vi "Choo Choo Test Bench.vi"() -> ()   [LabVIEW 2013]
doc: "This VI imlements the framework and scheduler for your robotics program. It should not be necessary to modify the framework. You are expected to add your code to the VIs called from Robot Main, the ones located in the Team Code within the project."
uses:
  <vilib>/Rock Robotics/WPI/Joystick/WPI_JoystickDeviceEnum.ctl
  <vilib>/Rock Robotics/SystemInterfaces/DIO/FPGA_DIOChannel.ctl
  <vilib>/Rock Robotics/SystemInterfaces/DIO/FPGA_DIOPWMChannel.ctl
  <vilib>/Rock Robotics/WPI/SafetyOutput/WPI_SafetyOutputConfigMenu.ctl
  <vilib>/Rock Robotics/SystemInterfaces/Typedef/FPGA_TypedefDigitalModule.ctl
  Competition Code/Robot Global Data.vi
  <vilib>/Rock Robotics/WPI/MotorControl/WPI_MotorControlOpen Jaguar.vi
  Competition Code/Choo Choo State.ctl
  <vilib>/Rock Robotics/WPI/DigitalInput/WPI_DigitalInputDevRef.ctl
  <vilib>/Rock Robotics/SystemInterfaces/Encoder/FPGA_EncoderIdx.ctl
  <vilib>/Rock Robotics/SystemInterfaces/Counter/FPGA_CounterCtrSystemIndex.ctl
  <vilib>/Rock Robotics/WPI/Encoder/WPI_EncoderType.ctl
  <vilib>/Rock Robotics/WPI/Encoder/WPI_EncoderDevRef.ctl
  <vilib>/Rock Robotics/WPI/PWM/WPI_PWMDeadband.ctl
  <vilib>/Rock Robotics/WPI/CAN/Jaguar/SubVIs/WPI_CANJaguar_ControlMode.ctl
  <vilib>/Rock Robotics/WPI/PWM/WPI_PWMTransform_ConPane.ctl
  <vilib>/Rock Robotics/WPI/MotorControl/WPI_MotorControlDeviceRef.ctl
  <vilib>/Rock Robotics/Network Tables/SD Write Number.vi
panel:
  in  "Finish":bool
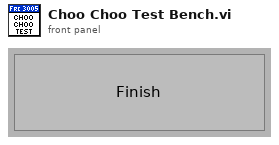
[diagram p1: front panel]
types:
  T1 = typedef "FPGA_TypedefDigitalModule.ctl" = enum16{"Digital Module 1", "Digital Module 2"}
  T2 = typedef "FPGA_DIOChannel.ctl" = enum8{"DIO 1", "DIO 2", "DIO 3", "DIO 4", "DIO 5", "DIO 6", "DIO 7", "DIO 8", "DIO 9", "DIO 10", "DIO 11", "DIO 12", "DIO 13", "DIO 14", "Invalid"}
  T3 = typedef "WPI_SafetyOutputConfigMenu.ctl" = enum16{"Enable", "Disable"}
  T4 = typedef "FPGA_DIOPWMChannel.ctl" = enum8{"PWM 1", "PWM 2", "PWM 3", "PWM 4", "PWM 5", "PWM 6", "PWM 7", "PWM 8", "PWM 9", "PWM 10", "Invalid"}
  T5 = typedef "WPI_MotorControlDeviceRef.ctl" = cluster{"DeviceStatus":errorcluster, "Type":enum16{"PWM", "CAN"}, "PWM":cluster{"Digital Module":T1, "PWM Channel":T4, "DeadBand":T6}, "CAN":cluster{"Device Number":u8, "Control Mode":T7, "Semaphore":T8, "Max Vout":dbl}, "Invert":bool, "TransformRef":T9, "InvTransformRef":T9}
  T6 = typedef "WPI_PWMDeadband.ctl" = cluster{"Name":string, "maxPositivePwm":i32, "minPositivePwm":i32, "centerPwm":i32, "maxNegativePwm":i32, "minNegativePwm":i32, "angularRange":u16}
  T7 = typedef "WPI_CANJaguar_ControlMode.ctl" = enum8{"Percent VBus", "Current", "Speed", "Position", "Voltage"}
  T8 = typedef "Semaphore RefNum" = refnum<k1>
  T9 = typedef "WPI_PWMTransform_ConPane.ctl" = refnum<vi>
  T10 = typedef "WPI_DigitalInputDevRef.ctl" = cluster{"DevStatus":errorcluster, "DIO Channel":T2, "Digital Module":T1}
  T11 = typedef "WPI_JoystickDeviceEnum.ctl" = enum16{"USB 1", "USB 2", "USB 3", "USB 4", "Kinect 1", "Kinect 2"}
  T12 = typedef "WPI_JoystickDevRef.ctl" = cluster{"Device":T11}
  T13 = typedef "WPI_EncoderDevRef.ctl" = cluster{"DevStatus":errorcluster, "EncoderIndex":T14, "CounterIndex":T15, "DistancePerCount":dbl, "Decoding Type":T16}
  T14 = typedef "FPGA_EncoderIdx.ctl" = enum8{"Enc 0", "Enc 1", "Enc 2", "Enc 3", "Invalid"}
  T15 = typedef "FPGA_CounterCtrSystemIndex.ctl" = enum8{"Ctr 0", "Ctr 1", "Ctr 2", "Ctr 3", "Ctr 4", "Ctr 5", "Ctr 6", "Ctr 7", "Invalid"}
  T16 = typedef "WPI_EncoderType.ctl" = enum16{"1x", "2x", "4x"}
  T17 = cluster{"Ball Detect":T10, "CC Switch":T10, "EncoderDevRef":T13, "MotorControlDevRef":T5}
  T18 = typedef "Choo Choo State.ctl" = enum16{"Idle", "Check For Ball", "Drive Motor", "Delay", "Check Status", "Stop Motor"}
  T19 = typedef "WPI_JoystickButtonState.ctl" = cluster{"Button 1":bool, "Button 2":bool, "Button 3":bool, "Button 4":bool, "Button 5":bool, "Button 6":bool, "Button 7":bool, "Button 8":bool, "Button 9":bool, "Button 10":bool, "Button 11":bool, "Button 12":bool}
  T20 = typedef "WPI_DriverStationRobotMode2.ctl" = enum16{"Autonomous Disabled", "Autonomous Enabled", "Teleop Disabled", "Teleop Enabled", "Timeout", "Finish", "Test Disabled", "Test Enabled"}
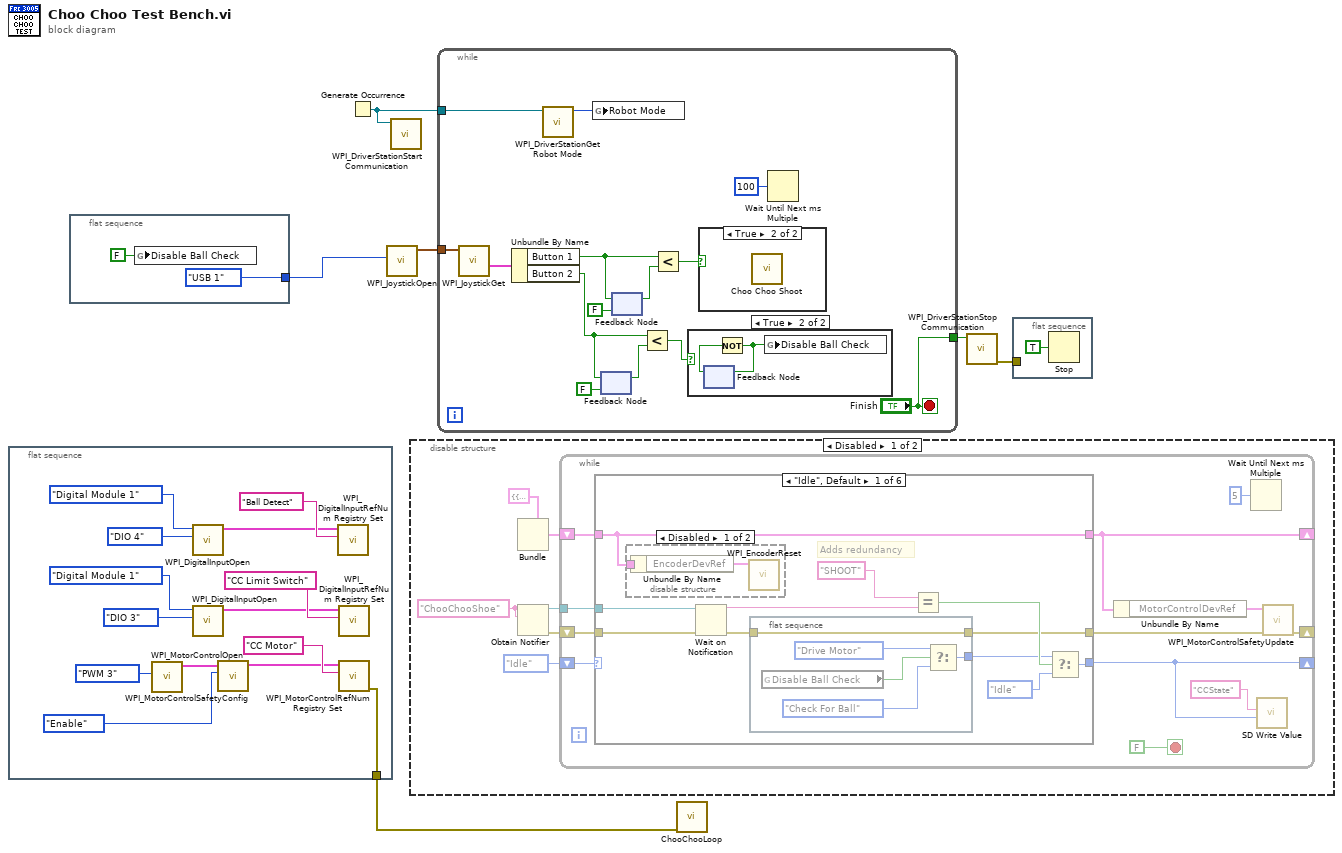
[diagram p0: block diagram]
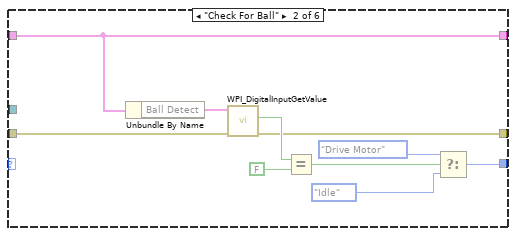
[diagram p3: hidden frame]
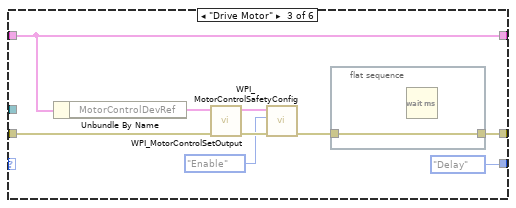
[diagram p4: hidden frame]
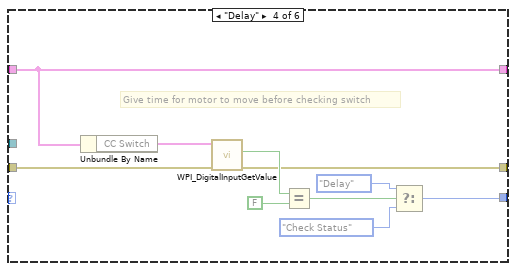
[diagram p5: hidden frame]
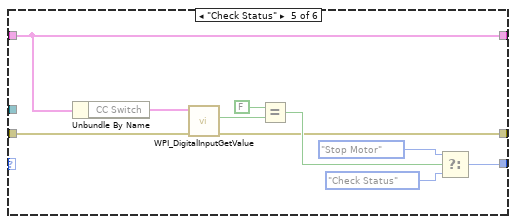
[diagram p6: hidden frame]
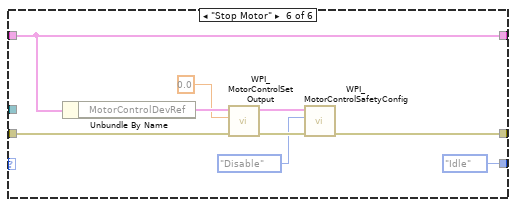
[diagram p7: hidden frame]
diagram:
  n1 = flat-sequence {
    tunnel: [w7] -> w1
    frame #0 {
      n2 = call-poly <vilib>:"WPI_MotorControlOpen.vi"("PWM Channel"=FPGA_DIOPWMChannel."PWM 3") -> ("MotorControlDeviceRef"=w17:T5)  [unwired: 9 in, 1 out]
      n3 = call <vilib>:"WPI_DigitalInputOpen.vi"("DIO Channel"=FPGA_DIOChannel."DIO 4", "Digital Module (Module 1)"=FPGA_TypedefDigitalModule."Digital Module 1") -> ("DigitalInputDevRef"=w10:T10)  [unwired: 8 in, 1 out]
      n4 = call <vilib>:"WPI_DigitalInputOpen.vi"("DIO Channel"=FPGA_DIOChannel."DIO 3", "Digital Module (Module 1)"=FPGA_TypedefDigitalModule."Digital Module 1") -> ("DigitalInputDevRef"=w9:T10)  [unwired: 8 in, 1 out]
      n5 = call <vilib>:"WPI_MotorControlSafetyConfig.vi"("mode"=WPI_SafetyOutputConfigMenu."Enable", "MotorControlDevRef"=w17) -> ("MotorControlDevRef"=w8:T5)  [unwired: 8 in, 1 out]
      n6 = call <vilib>:"WPI_DigitalInputRefNum Registry Set.vi"("refnum name"="Ball Detect", "DigitalInputDevRef"=w10) -> ()  [unwired: 8 in, 2 out]
      n7 = call <vilib>:"WPI_DigitalInputRefNum Registry Set.vi"("refnum name"="CC Limit Switch", "DigitalInputDevRef"=w9) -> ()  [unwired: 8 in, 2 out]
      n8 = call <vilib>:"WPI_MotorControlRefNum Registry Set.vi"("refnum name"="CC Motor", "MotorControlDevRef"=w8) -> ("error out"=w7:errorcluster)  [unwired: 8 in, 1 out]
    }
  }
  n9 = flat-sequence {
    tunnel: [WPI_JoystickDeviceEnum."USB 1" ("JoystickDevice")] -> w3
    frame #0 {
      n10 = global write "Robot Global Data.vi" "Disable Ball Check"(FALSE ("Disable Ball Check")) -> ()
    }
  }
  n11 = Generate Occurrence() -> (w2:refnum<k4>)
  n12 = call <vilib>:"WPI_JoystickOpen.vi"("JoystickDevice"=w3) -> ("JoystickDevRef"=w5:T12)  [unwired: 10 in]
  n13 = call <vilib>:"WPI_DriverStationStart Communication.vi"("occurrence"=w2) -> ()  [unwired: 11 out]
  n14 = disable-structure shown="Disabled" {
    frame Disabled {
      w26 = "ChooChooShoe" ("name (unnamed)")
      n15 = Bundle(cluster=T17 {"Ball Detect"={"DevStatus"={"status"=FALSE, "code"=0, "source"=""}, "DIO Channel"=enum."DIO 1", "Digital Module"=enum."Digital Module 1"}, "CC Switch"={"DevStatus"={"status"=FALSE, "code"=0, "source"=""}, "DIO Channel"=enum."DIO 1", "Digital Module"=enum."Digital Module 1"}, "EncoderDevRef"={"DevStatus"={"status"=FALSE, "code"=0, "source"=""}, "EncoderIndex"=enum."Enc 0", "CounterIndex"=enum."Ctr 0", "DistancePerCount"=0.0, "Decoding Type"=enum."1x"}, "MotorControlDevRef"={"DeviceStatus"={"status"=FALSE, "code"=0, "source"=""}, "Type"=enum."PWM", "PWM"={"Digital Module"=enum."Digital Module 1", "PWM Channel"=enum."PWM 1", "DeadBand"={"Name"="", "maxPositivePwm"=0, "minPositivePwm"=0, "centerPwm"=0, "maxNegativePwm"=0, "minNegativePwm"=0, "angularRange"=0}}, "CAN"={"Device Number"=0, "Control Mode"=enum."Percent VBus", "Semaphore"=refnum, "Max Vout"=0.0}, "Invert"=FALSE, "TransformRef"=refnum, "InvTransformRef"=refnum}}) -> (w28:T17)  [unwired: 3 in, 1 out]
      n16 = Obtain Notifier(name (unnamed)=w26, notification data type=w26) -> (notifier out=w25:refnum<notifier>, error out=w24:errorcluster)  [unwired: 2 in, 1 out]
      n17 = while {
        shift-right: [w31] -> _
        shift-left: w28 -> [w38]
        shift-right: [w29] -> _
        shift-left: Choo_Choo_State."Idle" -> [w37]
        tunnel: w25 -> [w36]
        shift-right: [w32] -> _
        shift-left: w24 -> [w35]
        stop <- FALSE stop-if-true
        n18 = case shown="\"Idle\", Default" w37 {
          tunnel: w38 -> [w45 w68 w78 w90 w100 w109]
          tunnel: [w45 w68 w78 w90 w100 w109] -> w31
          tunnel: w36 -> [w51 _ _ _ _ _]
          tunnel: [w47 w63 Choo_Choo_State."Delay" w85 w93 Choo_Choo_State."Idle"] -> w29
          tunnel: [w41 w59 w73 w81 w91 w103] -> w33
          tunnel: w35 -> [w46 w66 w75 w88 w92 w107]
          frame "Idle", Default {
            # "Adds redundancy"
            n19 = disable-structure shown="Disabled" {
              disable-tunnel: w45 -> [w58 _]
              frame Disabled {
                n20 = Unbundle By Name(w58) -> ("EncoderDevRef"=w57:T13)
                n21 = call <vilib>:"WPI_EncoderReset.vi"("EncoderDevRef"=w57) -> ()  [unwired: 9 in, 2 out]
              }
              frame Enabled {
              }
            }
            n22 = Wait on Notification(notifier=w51, error in (no error)=w46) -> (notification=w49:string, error out=w42:errorcluster)  [unwired: 2 in, 2 out]
            n23 = flat-sequence {
              tunnel: [w56] -> w43
              tunnel: w42 -> [w52]
              tunnel: [w52] -> w41
              frame #0 {
                n24 = global read "Robot Global Data.vi" "Disable Ball Check"() -> (w53:bool)
                n25 = Select(t=Choo_Choo_State."Drive Motor", s=w53, f=Choo_Choo_State."Check For Ball") -> (s? t:f=w56:T18)
              }
            }
            n26 = Equal?(x="SHOOT" ("name (unnamed)"), y=w49) -> (x = y?=w48:bool)
            n27 = Select(t=w43, s=w48, f=Choo_Choo_State."Idle") -> (s? t:f=w47:T18)
          }
          frame "Check For Ball" {
            n28 = Unbundle By Name(w68) -> ("Ball Detect"=w67:T10)
            n29 = call <vilib>:"WPI_DigitalInputGetValue.vi"("error in (no error)"=w66, "DigitalInputDevRef"=w67) -> ("error out"=w59:errorcluster, "Value"=w65:bool)  [unwired: 7 in, 1 out]
            n30 = Equal?(x=w65, y=FALSE ("x")) -> (x = y?=w62:bool)
            n31 = Select(t=Choo_Choo_State."Drive Motor", s=w62, f=Choo_Choo_State."Idle") -> (s? t:f=w63:T18)
          }
          frame "Drive Motor" {
            n32 = Unbundle By Name(w78) -> ("MotorControlDevRef"=w77:T5)
            n33 = call <vilib>:"WPI_MotorControlSetOutput.vi"("error in (no error)"=w75, "MotorControlDevRef"=w77) -> ("error out"=w72:errorcluster, "MotorControlDevRef"=w71:T5, "Output"=w76:dbl)  [unwired: 6 in, 1 out]
            n34 = call <vilib>:"WPI_MotorControlSafetyConfig.vi"("error in (no error)"=w72, "mode"=WPI_SafetyOutputConfigMenu."Enable", "MotorControlDevRef"=w71) -> ("error out"=w70:errorcluster)  [unwired: 7 in, 1 out]
            n35 = flat-sequence {
              tunnel: w70 -> [w79]
              tunnel: [w79] -> w73
              frame #0 {
                n36 = Wait (ms)() -> (milliseconds to wait=w80:u32)  [unwired: 1 out]
              }
            }
          }
          frame "Delay" {
            # "Give time for motor to move before checking switch"
            n37 = Unbundle By Name(w90) -> ("CC Switch"=w89:T10)
            n38 = call <vilib>:"WPI_DigitalInputGetValue.vi"("error in (no error)"=w88, "DigitalInputDevRef"=w89) -> ("error out"=w81:errorcluster, "Value"=w87:bool)  [unwired: 7 in, 1 out]
            n39 = Equal?(x=w87, y=FALSE ("x")) -> (x = y?=w84:bool)
            n40 = Select(t=Choo_Choo_State."Delay", s=w84, f=Choo_Choo_State."Check Status") -> (s? t:f=w85:T18)
          }
          frame "Check Status" {
            n41 = Unbundle By Name(w100) -> ("CC Switch"=w99:T10)
            n42 = call <vilib>:"WPI_DigitalInputGetValue.vi"("error in (no error)"=w92, "DigitalInputDevRef"=w99) -> ("error out"=w91:errorcluster, "Value"=w98:bool)  [unwired: 7 in, 1 out]
            n43 = Equal?(x=FALSE ("y"), y=w98) -> (x = y?=w94:bool)
            n44 = Select(t=Choo_Choo_State."Stop Motor", s=w94, f=Choo_Choo_State."Check Status") -> (s? t:f=w93:T18)
          }
          frame "Stop Motor" {
            n45 = Unbundle By Name(w109) -> ("MotorControlDevRef"=w108:T5)
            n46 = call <vilib>:"WPI_MotorControlSetOutput.vi"("error in (no error)"=w107, "Output"=0.0, "MotorControlDevRef"=w108) -> ("error out"=w104:errorcluster, "MotorControlDevRef"=w102:T5)  [unwired: 6 in, 1 out]
            n47 = call <vilib>:"WPI_MotorControlSafetyConfig.vi"("error in (no error)"=w104, "mode"=WPI_SafetyOutputConfigMenu."Disable", "MotorControlDevRef"=w102) -> ("error out"=w103:errorcluster)  [unwired: 7 in, 1 out]
          }
        }
        n48 = Unbundle By Name(w31) -> ("MotorControlDevRef"=w30:T5)
        n49 = Wait Until Next ms Multiple(millisecond multiple=u32 5 ("milliseconds to wait")) -> ()  [unwired: 1 out]
        n50 = call-poly <vilib>:"SD Write Value.vi"("Numeric"=w29, "Table Prefix"="CCState") -> ()  [unwired: 8 in, 2 out]
        n51 = call <vilib>:"WPI_MotorControlSafetyUpdate.vi"("error in (no error)"=w33, "MotorControlDevRef"=w30) -> ("error out"=w32:errorcluster)  [unwired: 8 in, 1 out]
      }
    }
    frame Enabled {
    }
  }
  n52 = while {
    tunnel: w5 -> [w122]
    tunnel: ["Finish"] -> w4
    tunnel: w2 -> [w110]
    stop <- "Finish" stop-if-true
    n53 = call <vilib>:"WPI_JoystickGet.vi"("JoystickDevRef"=w122) -> ("Buttons"=w121:T19)  [unwired: 4 in, 2 out]
    n54 = Unbundle By Name(w121) -> ("Button 1"=w114:bool, "Button 2"=w112:bool)
    n55 = call <vilib>:"WPI_DriverStationGet Robot Mode.vi"("DS Occurrence"=w110) -> ("Robot Mode"=w111:T20)  [unwired: 7 in, 3 out]
    n56 = global write "Robot Global Data.vi" "Robot Mode"(w111) -> ()
    n57 = feedback #1(FALSE) -> (w116:bool)
    n58 = feedback-in #1(w112) -> ()
    n59 = feedback-in #2(w114) -> ()
    n60 = feedback #2(FALSE) -> (w117:bool)
    n61 = Less?(x=w112, y=w116) -> (x < y?=w113:bool)
    n62 = Less?(x=w114, y=w117) -> (x < y?=w120:bool)
    n63 = case shown="True" w113 {
      frame False {
      }
      frame True {
        n64 = feedback #3() -> (w125:bool)  [unwired: 1 in]
        n65 = Not(x=w125) -> (.not. x?=w124:bool)
        n66 = feedback-in #3(w124) -> ()
        n67 = global write "Robot Global Data.vi" "Disable Ball Check"(w124) -> ()
      }
    }
    n68 = case shown="True" w120 {
      frame False {
      }
      frame True {
        n69 = call "Choo Choo Shoot.vi"() -> ()  [unwired: 11 in, 1 out]
      }
    }
    n70 = Wait Until Next ms Multiple(millisecond multiple=u32 100) -> ()  [unwired: 1 out]
  }
  n71 = call "ChooChooLoop.vi"("error in"=w1) -> ()  [unwired: 11 in]
  n72 = call <vilib>:"WPI_DriverStationStop Communication.vi"("StopCommunication"=w4) -> ("error out"=w6:errorcluster)  [unwired: 1 in, 9 out]
  n73 = flat-sequence {
    tunnel: w6 -> [_]
    frame #0 {
      n74 = Stop(stop? (T)=TRUE) -> ()
    }
  }
